vi "Open Local UDP Connection.vi"(8 "error in":errorcluster, 10 "Local Listening UDP Port":u16, 11 "Destination IP":string) -> (0 "Error out":errorcluster, 3 "Local UDP Connection ref":refnum<k16>)   [LabVIEW 2021, in "UDP Comms.lvlib"]
uses:
  UDP Comms.lvlib
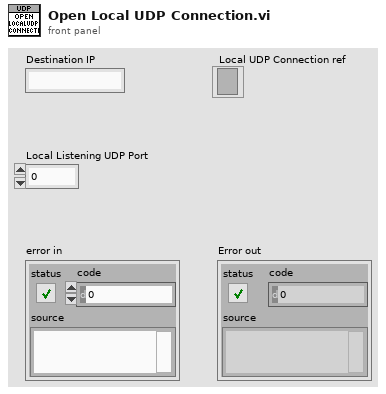
[diagram p1: front panel]
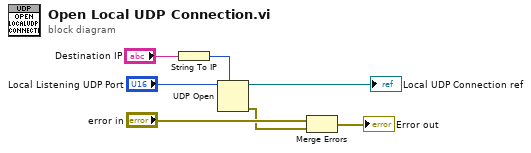
[diagram p0: block diagram]
diagram:
  n1 = String To IP(1:"Destination IP") -> (0:w1:u32)
  n2 = UDP Open(7:w1, 11:"Local Listening UDP Port") -> (port=→"Local UDP Connection ref":refnum<k16>, 0:w5:errorcluster)  [unwired: 3 in, 1 out]
  n3 = Merge Errors("error in", w5) -> (→"Error out":errorcluster)
